vi "GET_all_publishers.vi"() -> ()   [LabVIEW 2024, in "CV_RESTful_Lib.lvlib"]
uses:
  CV_RESTful_Lib.lvlib
  typedefs/local_publisher--cluster.ctl
  67a28660-369a-4700-940e-ce43c35547c4.vi
  <vilib>/addons/_JKI.lib/REST Client/classes/REST Client/REST Client.lvclass
  CV_Shared_Library/CV_Shared_Library.lvlib
  <vilib>/addons/_JKI.lib/Serialization/JSON/JKI JSON Serialization.lvlib
panel:
  out "size(s)":i32
  in  "stop":bool
  out "error out":errorcluster
  out "Array":T1[](array[typedef])
  out "name":string
  out "array with duplicates removed":i32[](array[numeric])
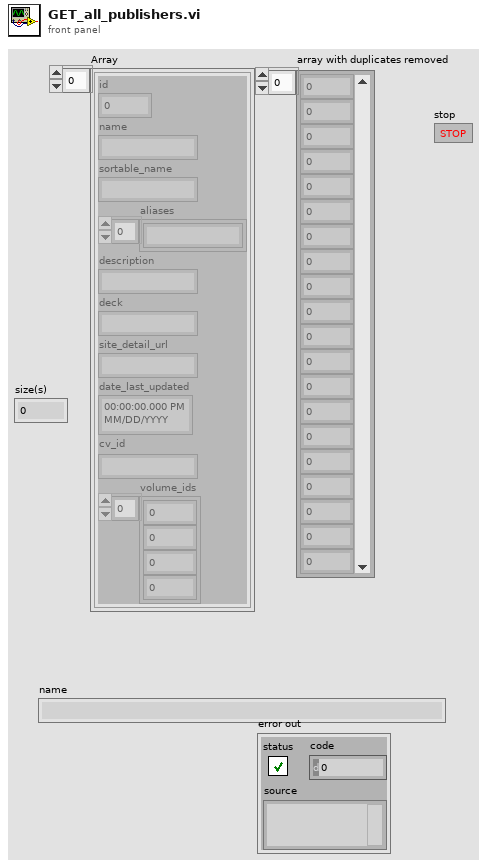
[diagram p1: front panel]
types:
  T1 = typedef "CV_RESTful_Lib.lvlib/local_publisher--cluster.ctl" = cluster{"id":i32, "name":string, "sortable_name":string, "aliases":string[], "description":string, "deck":string, "site_detail_url":string, "date_last_updated":timestamp, "cv_id":string, "volume_ids":i32[]}
  T2 = typedef "CV_RESTful_Lib.lvlib/local_volume--cluster.ctl" = cluster{"id":i32, "name":string, "sortable_name":string, "aliases":string[], "description":string, "site_detail_url":string, "count_of_issues":i32, "start_year":i32, "publisher_id":i32, "issue_ids":i32[], "date_last_updated":timestamp, "volume":i32, "cv_id":string, "volume type":T3}
  T3 = typedef "CV_Shared_Library.lvlib/volume.type--enum.ctl" = enum16{"Ongoing", "Limited Series", "Annual", "One Shot", "Reprint/Document", "Star Comics", "Epic Comics"}
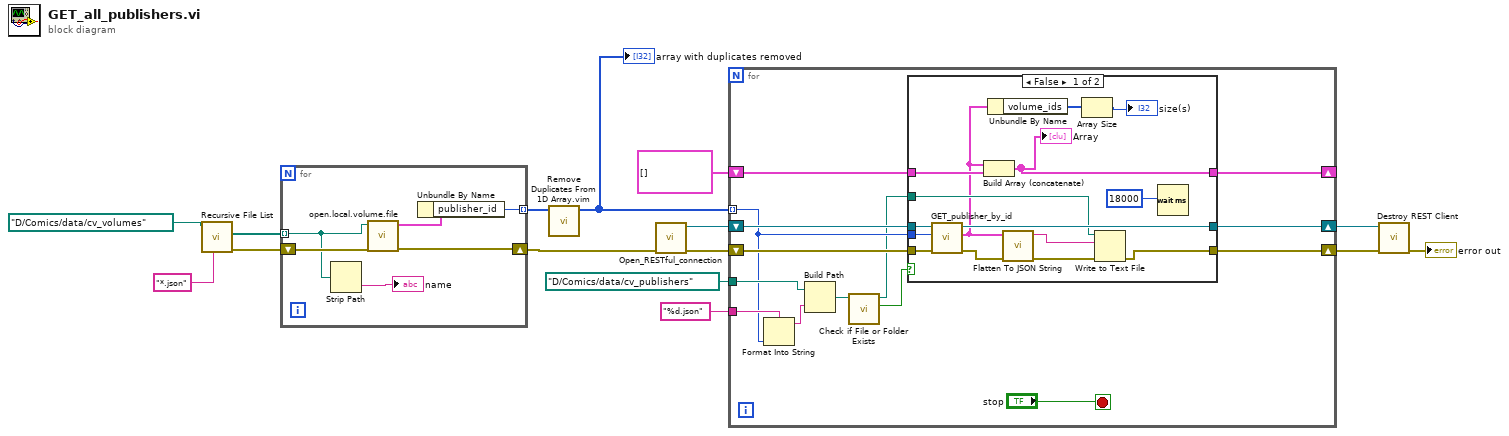
[diagram p0: block diagram]
diagram:
  n1 = call <vilib>:"Recursive File List.vi"("pattern"="*.json", "Folder Path"=path "D:/Comics/data/cv_volumes") -> ("error out"=w14:errorcluster, "All Files in Dir"=w12:path[])  [unwired: 5 in, 3 out]
  n2 = for {
    shift-right: [w18] -> w10
    shift-left: w14 -> [w21]
    tunnel: w12 -> [w17] mode=indexing
    tunnel: [w19] -> w11 mode=indexing
    n3 = Strip Path(path=w17) -> (name=→"name":string)  [unwired: 1 out]
    n4 = call "open.local.volume.file.vi"("error in (no error)"=w21, "volume json"=w17) -> ("error out"=w18:errorcluster, "volume"=w20:T2)  [unwired: 8 in]
    n5 = Unbundle By Name(w20) -> ("publisher_id"=w19:i32)
  }
  n6 = call "Remove Duplicates From 1D Array.vim"("array"=w11) -> ("array with duplicates removed"=w5:i32[])  [unwired: 10 in]
  "array with duplicates removed" <- w5
  n7 = call "Open_RESTful_connection.vi"("error in (no error)"=w10) -> ("error out"=w9:errorcluster, "REST Client out"=w8:refnum<class "REST Client.lvclass">)  [unwired: 9 in]
  n8 = for {
    shift-right: [w29] -> w7
    shift-left: w9 -> [w35]
    shift-right: [w33] -> w6
    shift-left: w8 -> [w34]
    tunnel: w5 -> [w25] mode=indexing
    shift-right: [w31] -> _
    shift-left: T1[] [] ("local volume") -> [w32]
    tunnel: "%d.json" ("format string") -> [w28]
    tunnel: path "D:/Comics/data/cv_publishers" -> [w26]
    stop <- "stop" stop-if-true
    n9 = Format Into String(format string=w28, w25) -> (resulting string=w27:string)  [unwired: 2 in, 1 out]
    n10 = Build Path(base path=w26, name or relative path=w27) -> (appended path=w24:path)
    n11 = call <vilib>:"Check if File or Folder Exists.vi"("path"=w24) -> ("file or folder exists?"=w22:bool, "dup path"=w23:path)  [unwired: 8 in, 1 out]
    n12 = case shown="False" w22 {
      tunnel: w35 -> [w50 w51]
      tunnel: w34 -> [w49 w52]
      tunnel: [w48 w52] -> w33
      tunnel: w32 -> [w47 w53]
      tunnel: [w46 w53] -> w31
      tunnel: [w42 w51] -> w29
      tunnel: w23 -> [w41 _]
      tunnel: w25 -> [w37 _]
      frame False {
        n13 = call "GET_publisher_by_id.vi"("error in (no error)"=w50, "publisher id"=w37, "REST Client in"=w49) -> ("error out"=w45:errorcluster, "local volume"=w40:T1, "REST Client out"=w48:refnum<class "REST Client.lvclass">)  [unwired: 6 in]
        n14 = Build Array (concatenate)(w40, w47) -> (w46:T1[])
        "Array" <- w46
        n15 = Unbundle By Name(w40) -> ("volume_ids"=w39:i32[])
        n16 = call <vilib>:"Flatten To JSON String.vi"("error in"=w45, "Variant"=w40) -> ("error out"=w44:errorcluster, "JSON String"=w43:string)  [unwired: 8 in]
        n17 = Array Size(array=w39) -> (size(s)=→"size(s)":i32)
        n18 = Write to Text File(file (use dialog)=w41, text=w43, error in=w44) -> (error out=w42:errorcluster)  [unwired: 1 in, 2 out]
        n19 = Wait (ms)(milliseconds to wait=u32 18000) -> ()  [unwired: 1 out]
      }
      frame True {
      }
    }
  }
  n20 = call-dynamic "Destroy REST Client.vi"("error in (no error)"=w7, "REST Client in"=w6) -> ("error out"=→"error out":errorcluster)  [unwired: 9 in]
